vi "auto_ir.vi"() -> ()   [LabVIEW 2012, in "BlockParty4150.lvrbt"]
uses:
  BlockParty4150.lvrbt
  <vilib>/NXT/Subs/LVHSConnector.ctl
  <vilib>/NXT/LegoClasses/BrickReference/BrickReference.lvclass
  <vilib>/NXT/Block Support/NXT_ButtonSelector.ctl
  <vilib>/NXT/HiTechnic/HiTechnic Controls/HiTechnic Port.ctl
  <vilib>/NXT/Block Support/NXT_InputPort.ctl
  <vilib>/NXT/Hardware/Plugins/Tetrix 180 deg Servo/Tetrix180ServoAddress.ctl
  <vilib>/NXT/Hardware/Plugins/Tetrix DC Motor/TetrixDCMotorAddress.ctl
  <vilib>/NXT/Dual Mode Library/Display/drawText.vi
  <vilib>/NXT/Dual Mode Library/Sound/Tone.vi
  <vilib>/NXT/Dual Mode Library/prims/inRangeAndCoerce/inRangeAndCoerce_int.vi
  <vilib>/NXT/Dual Mode Library/Display/drawNumber.vi
  <vilib>/NXT/NXTIO Xnodes/NXTIONodeSubVIs/TETRIX IO Move DC Motors.vi
  <vilib>/NXT/NXTIO Xnodes/NXTIONodeSubVIs/TETRIX IO Stop DC Motors.vi
  <vilib>/NXT/NXTIO Xnodes/NXTIONodeSubVIs/TETRIX IO Move Servos.vi
  <vilib>/NXT/Dual Mode Library/Waits/Wait_Num(msec).vi
  <vilib>/NXT/NXTIO Xnodes/AddressXNode/NXTIOAddress.xnode
  <vilib>/NXT/NXTIO Xnodes/NXTIOXNode/NXTIO.xnode
panel:
  out "Enabled":bool
  out "iter":i32
  out "NXT":T1
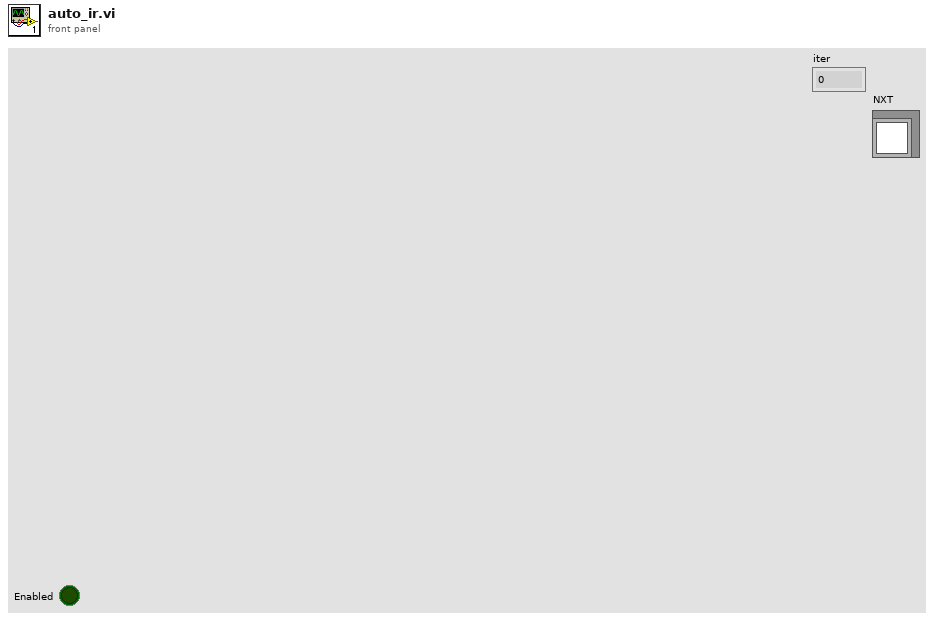
[diagram p1: front panel]
types:
  T1 = typedef "LVHSConnector.ctl" = refnum<class "BrickReference.lvclass">
  T2 = typedef "NXT_ButtonSelector.ctl" = u16
  T3 = typedef "Tetrix180ServoAddress.ctl" = i16
  T4 = typedef "TetrixDCMotorAddress.ctl" = i16
  T5 = typedef "HiTechnic Port.ctl" = cluster{"Port":T6, "MUX Port":u8}
  T6 = typedef "NXT_InputPort.ctl" = u8
  T7 = cluster{"Direction (0-9)":i16, "Signal Strength (Array)":u8[]}
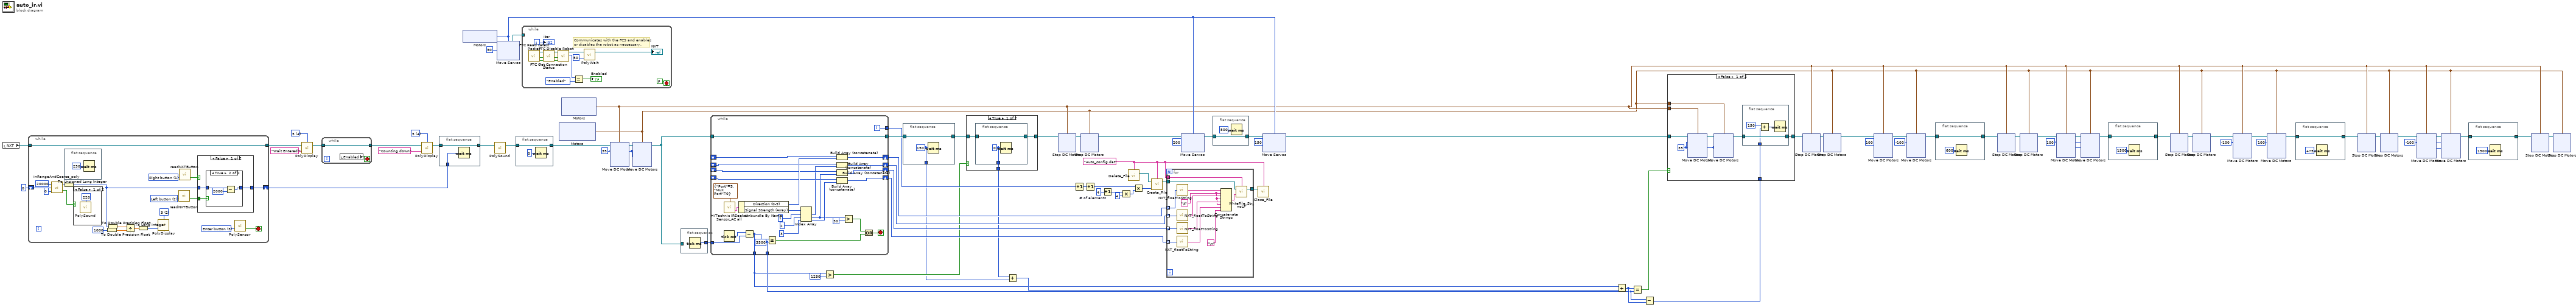
[diagram p0: block diagram]
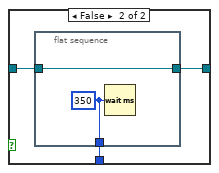
[diagram p2: hidden frame]
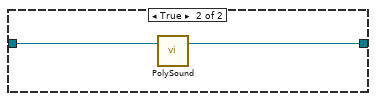
[diagram p3: hidden frame]
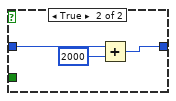
[diagram p6: hidden frame]
diagram:
  w17 = i8 -100 ("Power/Speed 1")
  w23 = i8 100 ("Power/Speed 1")
  w22 = i8 -100 ("Power/Speed 1")
  w29 = i8 100 ("Power/Speed 1")
  w35 = i8 -100 ("Power/Speed 1")
  w34 = i8 100 ("Power/Speed 1")
  w57 = 4  # # of elements
  w54 = "Auto_config.dat" ("Filename")
  w70 = i8 35 ("Power/Speed 1")
  w78 = i16 4 items=["1", "2", "3", "4", "5", "6", "7", "8"] ("Line")
  w79 = i16 4 items=["1", "2", "3", "4", "5", "6", "7", "8"] ("Line")
  n1 = local read "NXT"() -> (w72:T1)
  n2 = while {
    tunnel: [w107] -> w81
    tunnel: w72 -> [w107]
    shift-right: [w100] -> w82
    shift-left: u32 0 ("Power/Speed 1") -> [w93]
    stop <- w105 stop-if-true
    w99 = i16 2 items=["1", "2", "3", "4", "5", "6", "7", "8"] ("Line")
    w102 = T2 1 items=["Enter button"=3, "Left button"=2, "Right button"=1] ("Button (Enter button)")
    w101 = T2 2 items=["Enter button"=3, "Left button"=2, "Right button"=1] ("Button (Enter button)")
    w106 = T2 3 items=["Enter button"=3, "Left button"=2, "Right button"=1] ("Button (Enter button)")
    n3 = call-poly <vilib>:"inRangeAndCoerce_poly.vi"("lower limit"=0, "x"=w93, "upper limit"=20000) -> ("In Range?"=w88:bool, "coerced(x)"=w90:i32)
    n4 = To Unsigned Long Integer(number=w90) -> (unsigned 32bit integer=w89:u32)
    n5 = flat-sequence {
      frame #0 {
        n6 = Wait (ms)(milliseconds to wait=u32 250) -> ()  [unwired: 1 out]
      }
    }
    n7 = case shown="False" w88 {
      frame False {
        n8 = call-poly <vilib>:"PolySound.vi"("Tone (440 Hz)"=u16 220) -> ()  [unwired: 3 in, 1 out]
      }
      frame True {
      }
    }
    n9 = To Double Precision Float(number=u32 1000 ("Power/Speed 1")) -> (double precision float=w94:dbl)
    n10 = To Double Precision Float(number=w89) -> (double precision float=w96:dbl)
    n11 = Divide(x=w96, y=w94) -> (x/y=w97:dbl)
    n12 = To Long Integer(number=w97) -> (32bit integer=w95:i32)
    n13 = call-poly <vilib>:"PolyDisplay.vi"("number"=w95, "Line"=w99) -> ()  [unwired: 2 in, 1 out]
    n14 = call <vilib>:"readNXTButton.vi"("Button (Enter button)"=w101) -> ("Yes/No"=w104:bool)  [unwired: 2 in, 1 out]
    n15 = call <vilib>:"readNXTButton.vi"("Button (Enter button)"=w102) -> ("Yes/No"=w103:bool)  [unwired: 2 in, 1 out]
    n16 = case shown="False" w103 {
      tunnel: w104 -> [w112 _]
      tunnel: [w111 w118] -> w100
      tunnel: w89 -> [w110 w119]
      frame False {
        n17 = case shown="True" w112 {
          tunnel: [w113 w115] -> w111
          tunnel: w110 -> [w113 w116]
          frame False {
          }
          frame True {
            n18 = Subtract(x=w116, y=u32 2000) -> (x-y=w115:u32)
          }
        }
      }
      frame True {
        n19 = Add(x=w119, y=u32 2000) -> (x+y=w118:u32)
      }
    }
    n20 = call-poly <vilib>:"PolySensor.vi"("Button (Enter button)"=w106) -> ("Yes/No"=w105:bool)  [unwired: 2 in, 1 out]
  }
  n21 = call-poly <vilib>:"PolyDisplay.vi"("Text"="Wait Entered!", "NXT"=w81, "Line"=w79) -> ("NXT"=w74:T1)  [unwired: 1 in]
  n22 = while {
    tunnel: [w120] -> w73
    tunnel: w74 -> [w120]
    stop <- w121 stop-if-true
    n23 = local read "Enabled"() -> (w121:bool)
  }
  n24 = call-poly <vilib>:"PolyDisplay.vi"("Text"="Counting down", "NXT"=w73, "Line"=w78) -> ("NXT"=w76:T1)  [unwired: 1 in]
  n25 = flat-sequence {
    tunnel: w76 -> [w123]
    tunnel: [w123] -> w84
    tunnel: w82 -> [w122]
    frame #0 {
      n26 = Wait (ms)(milliseconds to wait=w122) -> ()  [unwired: 1 out]
    }
  }
  n27 = xnode "Motors"() -> ("Motor"=w85:T3)
  n28 = call-poly <vilib>:"PolySound.vi"("NXT"=w84) -> ("NXT"=w75:T1)  [unwired: 3 in]
  n29 = xnode "Move Servos"("Position 1"=u8 30, "Servos"=w85) -> ("NXT"=w86:T1)  [unwired: 1 in]
  n30 = flat-sequence {
    tunnel: w75 -> [w125]
    tunnel: [w125] -> w67
    frame #0 {
      n31 = Wait (ms)(milliseconds to wait=u32 0) -> ()  [unwired: 1 out]
    }
  }
  n32 = while {
    tunnel: w86 -> [_]
    i -> [w127]
    stop <- FALSE stop-if-true
    # "Communicates with the FCS and enables \nor disables the robot as neccessary."
    n33 = call <vilib>:"FTC Read Latest Packet.vi"() -> ("Packet Received?"=w137:bool, "Stopped?"=w136:bool, "NXT"=w139:T1)  [unwired: 6 in, 3 out]
    n34 = call <vilib>:"FTC Get Connection Status.vi"("Packet Received?"=w137, "Stopped?"=w136, "NXT"=w139) -> ("Online?"=w129:bool, "Stopped?"=w130:bool, "NXT"=w138:T1)  [unwired: 5 in]
    n35 = call <vilib>:"FTC Disable Robot.vi"("Online?"=w129, "Stopped?"=w130, "NXT"=w138) -> ("Enabled?"=w133:enum16{"Disabled", "Enabled"}, "NXT"=w135:T1)  [unwired: 3 in]
    n36 = Equal?(x=w133, y=enum16{"Disabled", "Enabled"}."Enabled") -> (x = y?=→"Enabled":bool)
    n37 = call-poly <vilib>:"PolyWait.vi"("Time (100 msec)"=u32 50 ("Time (msec)"), "NXT"=w135) -> ("NXT"=→"NXT":T1)  [unwired: 2 in]
    "iter" <- w127
  }
  n38 = xnode "Motors"() -> ("Motor"=w63:cluster{"TetrixDCMotor":T4, "TetrixDCMotor":T4})
  n39 = xnode "Motors"() -> ("Motor"=w64:cluster{"TetrixDCMotor":T4, "TetrixDCMotor":T4})
  n40 = xnode "Move DC Motors"("Power/Speed 2"=w70, "Power/Speed 1"=w70, "Motors"=w64, "NXT"=w67) -> ("NXT"=w71:T1)
  n41 = xnode "Move DC Motors"("Power/Speed 2"=w70, "Power/Speed 1"=w70, "Motors"=w63, "NXT"=w71) -> ("NXT"=w68:T1)
  n42 = flat-sequence {
    tunnel: [w140] -> w66
    tunnel: w68 -> [_]
    frame #0 {
      n43 = Tick Count (ms)() -> (millisecond timer value=w140:u32)
    }
  }
  n44 = while {
    tunnel: [w167] -> w10
    shift-right: [w166] -> w51
    shift-left: _ -> [w165]
    shift-right: [w163] -> w50
    shift-left: _ -> [w164]
    shift-right: [w152] -> w49
    shift-left: _ -> [w155]
    shift-right: [w151] -> w48
    shift-left: _ -> [w154]
    tunnel: w68 -> [w150]
    tunnel: [w150] -> w65
    tunnel: w66 -> [w143]
    tunnel: [w142] -> w1
    tunnel: [w141] -> w7
    i -> [w167]
    stop <- w147 stop-if-true
    w141 = u32 3500 ("y")
    n45 = Tick Count (ms)() -> (millisecond timer value=w168:u32)
    n46 = call <vilib>:"HiTechnic IRSeeker Sensor_AC all.vi"("Port/MUX"=T5 {"Port"=3, "MUX Port"=0}) -> ("All Info"=w162:T7)  [unwired: 2 in, 1 out]
    n47 = Unbundle By Name(w162) -> ("Direction (0-9)"=w158:i16, "Signal Strength (Array)"=w161:u8[])
    n48 = Subtract(x=w168, y=w143) -> (x-y=w142:u32)
    n49 = Greater Or Equal?(x=w142, y=w141) -> (x >= y?=w145:bool)
    n50 = Index Array(array=w161, index #1=1 ("index"), index #2=2 ("index"), index #3=3 ("index")) -> (element #1=w149:u8, element #2=w144:u8, element #3=w153:u8)
    n51 = Build Array (concatenate)(w165, w158) -> (w166:i16[])
    n52 = Build Array (concatenate)(w164, w149) -> (w163:u8[])
    n53 = Build Array (concatenate)(w155, w144) -> (w152:u8[])
    n54 = Build Array (concatenate)(w154, w153) -> (w151:u8[])
    n55 = Greater?(x=w144, y=u8 30) -> (0:w146:bool)
    n56 = Or(x=w146, y=w145) -> (x .or. y?=w147:bool)
  }
  n57 = Greater?(x=w1, y=u32 1250) -> (0:w5:bool)
  n58 = flat-sequence {
    tunnel: [w170] -> w9
    tunnel: w65 -> [w170]
    tunnel: [w169] -> w2
    frame #0 {
      w169 = u32 150 ("milliseconds to wait")
      n59 = Wait (ms)(milliseconds to wait=w169) -> ()  [unwired: 1 out]
    }
  }
  n60 = case shown="True" w5 {
    tunnel: w9 -> [w173 w178]
    tunnel: [w172 w177] -> w8
    tunnel: [w171 w176] -> w4
    frame True {
      n61 = flat-sequence {
        tunnel: [w175] -> w171
        tunnel: [w174] -> w172
        tunnel: w173 -> [w174]
        frame #0 {
          w175 = u32 0 ("milliseconds to wait")
          n62 = Wait (ms)(milliseconds to wait=w175) -> ()  [unwired: 1 out]
        }
      }
    }
    frame False {
      n63 = flat-sequence {
        tunnel: [w180] -> w176
        tunnel: [w179] -> w177
        tunnel: w178 -> [w179]
        frame #0 {
          w180 = u32 350 ("milliseconds to wait")
          n64 = Wait (ms)(milliseconds to wait=w180) -> ()  [unwired: 1 out]
        }
      }
    }
  }
  n65 = Add(x=w4, y=w2) -> (x+y=w3:u32)
  n66 = xnode "Stop DC Motors"("Motors"=w64, "NXT"=w8) -> ("NXT"=w69:T1)
  n67 = Increment(x=w10) -> (x+1=w55:i32)
  n68 = xnode "Stop DC Motors"("Motors"=w63, "NXT"=w69) -> ("NXT"=w42:T1)
  n69 = Increment(x=w55) -> (x+1=w61:i32)
  n70 = Increment(x=w57) -> (x+1=w58:i32)
  n71 = Multiply(x=w58, y=u32 4) -> (x*y=w59:u32)
  n72 = call <vilib>:"Delete_File.vi"("Filename"=w54) -> ("NXT"=w62:T1)  [unwired: 3 in]
  n73 = Multiply(x=w61, y=w59) -> (x*y=w52:u32)
  n74 = call <vilib>:"Create_File.vi"("File Size (256)"=w52, "NXT"=w62, "Filename"=w54) -> ("NXT"=w53:T1)  [unwired: 1 out]
  n75 = for {
    tunnel: w54 -> [w194]
    tunnel: w53 -> [w193]
    tunnel: [w192] -> w56
    tunnel: w51 -> [w191] mode=indexing
    tunnel: w50 -> [w189] mode=indexing
    tunnel: w49 -> [w182] mode=indexing
    tunnel: w48 -> [w181] mode=indexing
    w185 = "\t" ("string")
    n76 = call <vilib>:"NXT_floatToString.vi"("number"=w191) -> ("string"=w188:string)
    n77 = call <vilib>:"NXT_floatToString.vi"("number"=w189) -> ("string"=w187:string)
    n78 = call <vilib>:"NXT_floatToString.vi"("number"=w182) -> ("string"=w186:string)
    n79 = call <vilib>:"NXT_floatToString.vi"("number"=w181) -> ("string"=w184:string)
    n80 = Concatenate Strings(w188, w185, w187, w185, w186, w185, w184, "\n") -> (w190:string)
    n81 = call <vilib>:"WriteFile_Str_noLF.vi"("String"=w190, "NXT"=w193, "Filename"=w194) -> ("NXT"=w192:T1)  [unwired: 1 in]
  }
  n82 = xnode "Move Servos"("Position 1"=u8 200, "Servos"=w85, "NXT"=w42) -> ("NXT"=w46:T1)
  n83 = flat-sequence {
    tunnel: [w195] -> w44
    tunnel: w46 -> [w195]
    frame #0 {
      n84 = Wait (ms)(milliseconds to wait=u32 500) -> ()  [unwired: 1 out]
    }
  }
  n85 = call <vilib>:"Close_File.vi"("NXT"=w56, "Filename"=w54) -> ()  [unwired: 2 in, 1 out]
  n86 = xnode "Move Servos"("Position 1"=u8 150, "Servos"=w85, "NXT"=w44) -> ("NXT"=w43:T1)
  n87 = Add(x=w1, y=w3) -> (x+y=w40:u32)
  n88 = Equal?(x=w40, y=w7) -> (x = y?=w41:bool)
  n89 = Subtract(x=w7, y=w40) -> (x-y=w39:u32)
  n90 = case shown="False" w41 {
    tunnel: w43 -> [w204 w230]
    tunnel: [w201 w229] -> w37
    tunnel: w64 -> [w200 _]
    tunnel: w63 -> [w199 _]
    tunnel: w39 -> [w198 _]
    frame False {
      w197 = i8 35 ("Power/Speed 1")
      n91 = xnode "Move DC Motors"("Power/Speed 2"=w197, "Power/Speed 1"=w197, "Motors"=w200, "NXT"=w204) -> ("NXT"=w203:T1)
      n92 = xnode "Move DC Motors"("Power/Speed 2"=w197, "Power/Speed 1"=w197, "Motors"=w199, "NXT"=w203) -> ("NXT"=w202:T1)
      n93 = flat-sequence {
        tunnel: [w208] -> w201
        tunnel: w202 -> [w208]
        tunnel: w198 -> [w205]
        frame #0 {
          n94 = Add(x=u32 150, y=w205) -> (x+y=w207:u32)
          n95 = Wait (ms)(milliseconds to wait=w207) -> ()  [unwired: 1 out]
        }
      }
    }
    frame True {
      n96 = call-poly <vilib>:"PolySound.vi"("NXT"=w230) -> ("NXT"=w229:T1)  [unwired: 3 in]
    }
  }
  n97 = xnode "Stop DC Motors"("Motors"=w64, "NXT"=w37) -> ("NXT"=w38:T1)
  n98 = xnode "Stop DC Motors"("Motors"=w63, "NXT"=w38) -> ("NXT"=w36:T1)
  n99 = xnode "Move DC Motors"("Power/Speed 2"=w34, "Power/Speed 1"=w34, "Motors"=w64, "NXT"=w36) -> ("NXT"=w33:T1)
  n100 = xnode "Move DC Motors"("Power/Speed 2"=w35, "Power/Speed 1"=w35, "Motors"=w63, "NXT"=w33) -> ("NXT"=w30:T1)
  n101 = flat-sequence {
    tunnel: [w231] -> w32
    tunnel: w30 -> [w231]
    frame #0 {
      n102 = Wait (ms)(milliseconds to wait=u32 600) -> ()  [unwired: 1 out]
    }
  }
  n103 = xnode "Stop DC Motors"("Motors"=w64, "NXT"=w32) -> ("NXT"=w31:T1)
  n104 = xnode "Stop DC Motors"("Motors"=w63, "NXT"=w31) -> ("NXT"=w24:T1)
  n105 = xnode "Move DC Motors"("Power/Speed 2"=w29, "Power/Speed 1"=w29, "Motors"=w64, "NXT"=w24) -> ("NXT"=w28:T1)
  n106 = xnode "Move DC Motors"("Power/Speed 2"=w29, "Power/Speed 1"=w29, "Motors"=w63, "NXT"=w28) -> ("NXT"=w25:T1)
  n107 = flat-sequence {
    tunnel: [w233] -> w27
    tunnel: w25 -> [w233]
    frame #0 {
      n108 = Wait (ms)(milliseconds to wait=u32 1500) -> ()  [unwired: 1 out]
    }
  }
  n109 = xnode "Stop DC Motors"("Motors"=w64, "NXT"=w27) -> ("NXT"=w26:T1)
  n110 = xnode "Stop DC Motors"("Motors"=w63, "NXT"=w26) -> ("NXT"=w11:T1)
  n111 = xnode "Move DC Motors"("Power/Speed 2"=w22, "Power/Speed 1"=w22, "Motors"=w64, "NXT"=w11) -> ("NXT"=w21:T1)
  n112 = xnode "Move DC Motors"("Power/Speed 2"=w23, "Power/Speed 1"=w23, "Motors"=w63, "NXT"=w21) -> ("NXT"=w18:T1)
  n113 = flat-sequence {
    tunnel: [w235] -> w20
    tunnel: w18 -> [w235]
    frame #0 {
      n114 = Wait (ms)(milliseconds to wait=u32 475) -> ()  [unwired: 1 out]
    }
  }
  n115 = xnode "Stop DC Motors"("Motors"=w64, "NXT"=w20) -> ("NXT"=w19:T1)
  n116 = xnode "Stop DC Motors"("Motors"=w63, "NXT"=w19) -> ("NXT"=w12:T1)
  n117 = xnode "Move DC Motors"("Power/Speed 2"=w17, "Power/Speed 1"=w17, "Motors"=w64, "NXT"=w12) -> ("NXT"=w16:T1)
  n118 = xnode "Move DC Motors"("Power/Speed 2"=w17, "Power/Speed 1"=w17, "Motors"=w63, "NXT"=w16) -> ("NXT"=w13:T1)
  n119 = flat-sequence {
    tunnel: [w237] -> w15
    tunnel: w13 -> [w237]
    frame #0 {
      n120 = Wait (ms)(milliseconds to wait=u32 1500) -> ()  [unwired: 1 out]
    }
  }
  n121 = xnode "Stop DC Motors"("Motors"=w64, "NXT"=w15) -> ("NXT"=w14:T1)
  n122 = xnode "Stop DC Motors"("Motors"=w63, "NXT"=w14) -> ()  [unwired: 1 out]
